vi "F to C converter.vi"(10 "Boolean":bool, 11 "Temperature (F)":dbl) -> (3 "Numeric":dbl)   [LabVIEW 2018]
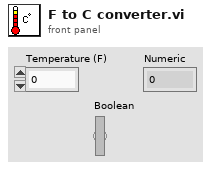
[diagram p1: front panel]
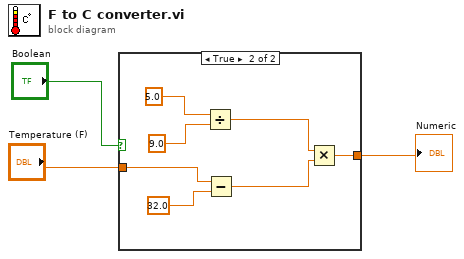
[diagram p0: block diagram]
diagram:
  n1 = case shown="True" "Boolean" {
    tunnel: [w4 w11] -> w3
    tunnel: "Temperature (F)" -> [w4 w6]
    frame False {
    }
    frame True {
      n2 = Divide(x=5.0, y=9.0) -> (x/y=w10:dbl)
      n3 = Subtract(x=w6, y=32.0) -> (x-y=w7:dbl)
      n4 = Multiply(x=w10, y=w7) -> (x*y=w11:dbl)
    }
  }
  "Numeric" <- w3
